vi "Export.vi"(8 "error in (no error)":errorcluster, 10 "IExporter":refnum<class "IExporter.lvclass">, 11 "CDependencyList in":refnum<class "CDependencyList.lvclass">) -> (0 "error out":errorcluster, 3 "CDependencyList out":refnum<class "CDependencyList.lvclass">)   [LabVIEW 2020, in "DependencyInspection.lvlib" / "CDependencyList.lvclass"]
uses:
  CDependencyList.lvclass
  obj/Addons/ExtensionInterfaces.lvlibp/IExporter/IExporter.lvclass
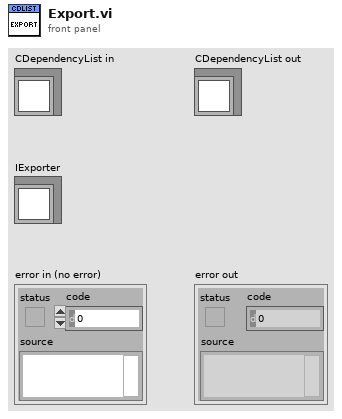
[diagram p1: front panel]
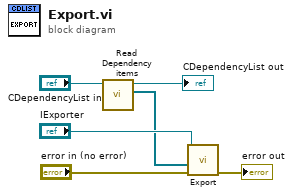
[diagram p0: block diagram]
diagram:
  n1 = call-dynamic "Read Dependency items.vi"("CDependencyList in"="CDependencyList in") -> ("Dependency items"=w3:refnum<class "ILabVIEWItem.lvclass">[], "CDependencyList out"=→"CDependencyList out":refnum<class "CDependencyList.lvclass">)  [unwired: 9 in]
  n2 = call-dynamic "Export.vi"("error in (no error)"="error in (no error)", "Items"=w3, "IExporter in"="IExporter") -> ("error out"=→"error out":errorcluster)  [unwired: 7 in, 1 out]
